vi "Test Async Handler Error Handled by Error Handler.vi"(8 "error in (no error)":errorcluster, 11 "Test Case In":refnum<class "Async Handling Test.lvclass">) -> (0 "error out":errorcluster, 3 "Test Case Out":refnum<class "Async Handling Test.lvclass">)   [LabVIEW 2020, in "Async Handling Test.lvclass"]
uses:
  Async Handling Test.lvclass
  C:/Program Files (x86)/National Instruments/LabVIEW 2020/vi.lib/Astemes/LUnit/Test Case.lvclass
  Mock Async Handler Process/Mock Async Handler Process.lvclass
  C:/Git/astemes-triarc-framework/source/Framework/Process/Process.lvclass
  source/Framework Test Suite/Mock Error Handler/Mock Error Handler.lvclass
  C:/Git/astemes-triarc-framework/source/Framework/Error Handler Interface/Error Handler Interface.lvclass
  source/Framework/Process/Process.lvclass/Process.ctl
  <vilib>/Astemes/LUnit/Test Case.lvclass/Test Case.ctl
  01074fa8-ee8a-411d-bc8b-fc92c4f90959.vi
  source/Framework/Process/Protected/Messaging/Send Message.vi
  source/Framework/Process/Public/Lifecycle/Get Lifecycle State.vi
  source/Framework/Process/Private/SubVIs/Wait for finish.vi
  source/Framework/Process/Private/SubVIs/Set Lifecycle State.vi
  <vilib>/Astemes/LUnit/Palette/Pass.vi
  <vilib>/Astemes/LUnit/Palette/Fail.vi
  <vilib>/Astemes/LUnit/Compare Variants.vi
  <vilib>/Astemes/LUnit/Describe Comparison.vi
  <vilib>/Astemes/LUnit/Set Assertion Type.vi
  source/Framework/Process/Private/SubVIs/Handle Debug Data.vi
  <vilib>/Utility/error.llb/Clear Errors.vi
  <vilib>/Astemes/LUnit/Add test result.vi
  <vilib>/Astemes/LUnit/Variant to string.vi
  source/Framework/Logging/Log Debug.vi
  <vilib>/AdvancedString/1D String Array to Delimited String.vi
  <vilib>/Utility/High Resolution Relative Seconds.vi
  <vilib>/Astemes/LUnit/LUnit Record Assertion Result.vi
  <vilib>/Astemes/LUnit/LUnit Aggregate Assertion Results.vi
  <vilib>/Astemes/LUnit/Method Result/LUnit Merge Status.vi
  <vilib>/Astemes/LUnit/LUnit Concatenate result strings.vi
  <vilib>/Utility/error.llb/Error Cluster From Error Code.vi
  source/Framework/Process/Public/Read Name.vi
  <vilib>/Utility/Data Type/Get Type Information.vi
  <vilib>/Utility/LVClass/Get LV Class Name.vi
  source/Framework/Process/Process.lvclass
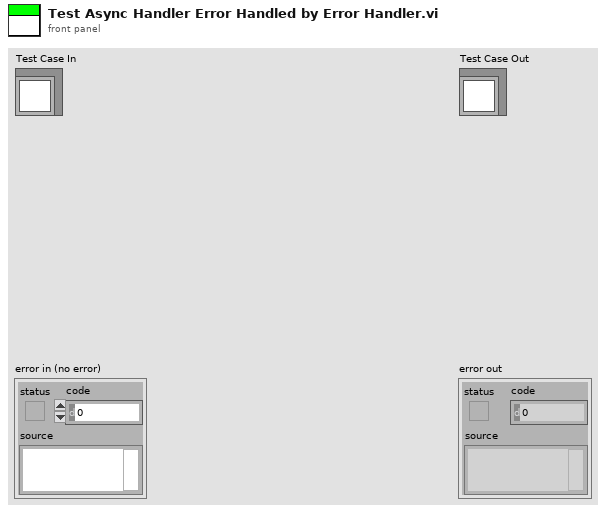
[diagram p1: front panel]
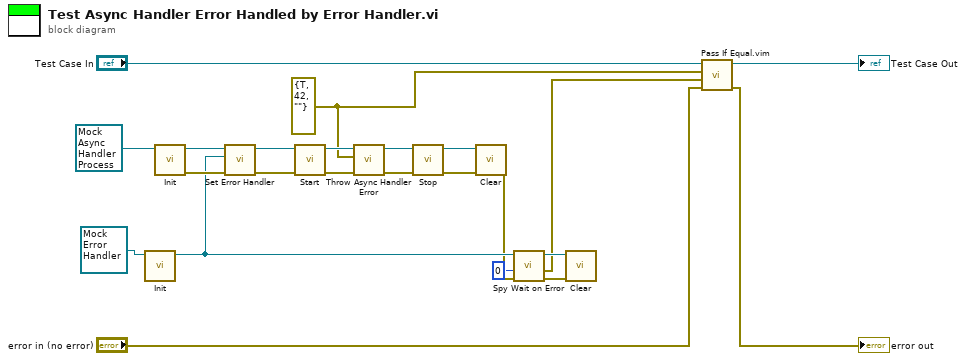
[diagram p0: block diagram]
diagram:
  w2 = errorcluster {"status"=TRUE, "code"=42, "source"=""} ("Error")
  n1 = call-dynamic "Init.vi"("Mock Error Handler In"=refnum<class "Mock Error Handler.lvclass"> refnum ("Mock Error Handler.lvclass")) -> ("Mock Error Handler Out"=w7:refnum<class "Mock Error Handler.lvclass">)  [unwired: 9 in, 1 out]
  n2 = call-dynamic "Init.vi"("Process In"=refnum<class "Mock Async Handler Process.lvclass"> refnum ("Mock Async Handler Process.lvclass")) -> ("error out"=w19:errorcluster, "Process Out"=w14:refnum<class "Mock Async Handler Process.lvclass">)  [unwired: 9 in]
  n3 = call "Set Error Handler.vi"("error in (no error)"=w19, "Error Handler"=w7, "Process In"=w14) -> ("error out"=w15:errorcluster, "Process Out"=w13:refnum<class "Mock Async Handler Process.lvclass">)  [unwired: 7 in]
  n4 = call "Start.vi"("error in (no error)"=w15, "Process In"=w13) -> ("error out"=w18:errorcluster, "Process Out"=w9:refnum<class "Mock Async Handler Process.lvclass">)  [unwired: 7 in, 1 out]
  n5 = call "Throw Async Handler Error.vi"("error in (no error)"=w18, "Error"=w2, "Mock Async Handler Process in"=w9) -> ("error out"=w12:errorcluster, "Mock Async Handler Process out"=w11:refnum<class "Mock Async Handler Process.lvclass">)  [unwired: 7 in]
  n6 = call "Stop.vi"("error in (no error)"=w12, "Process In"=w11) -> ("error out"=w16:errorcluster, "Process Out"=w17:refnum<class "Mock Async Handler Process.lvclass">)  [unwired: 7 in, 1 out]
  n7 = call-dynamic "Clear.vi"("error in (no error)"=w16, "Process In"=w17) -> ("error out"=w5:errorcluster)  [unwired: 9 in]
  n8 = call "Spy Wait on Error.vi"("error in (no error)"=w5, "timeout in ms (-1)"=0, "Mock Error Handler In"=w7) -> ("error out"=w4:errorcluster, "Errors"=w3:errorcluster, "Mock Error Handler Out"=w6:refnum<class "Mock Error Handler.lvclass">)  [unwired: 4 in, 2 out]
  n9 = call-dynamic "Clear.vi"("error in (no error)"=w4, "Mock Process In"=w6) -> ()  [unwired: 9 in, 1 out]
  n10 = call "Pass If Equal.vim"("error in (no error)"="error in (no error)", "Actual"=w3, "Expected"=w2, "LUnit Test Case In"="Test Case In") -> ("error out"=→"error out":errorcluster, "LUnit Test Case Out"=→"Test Case Out":refnum<class "Async Handling Test.lvclass">)  [unwired: 6 in]
